vi "Initialize.vi"(6 "Actor Name":string, 7 "Host Name":string, 8 "error in (no error)":errorcluster, 11 "Message Broker":refnum<class "Message Broker Interface Ref.lvclass">) -> (0 "error out":errorcluster, 3 "User Interface out":refnum<class "User Interface.lvclass">)   [LabVIEW 2016, in "CLD Exam - ATM.lvlib" / "User Interface.lvclass"]
uses:
  User Interface.lvclass
  D:/Repos/Stream/software/Mediator/Classes/Mediated Actor/Mediated Actor.lvclass
  Mediator/Classes/Message Broker Interface Ref/Message Broker Interface Ref.lvclass
  D:/Repos/Stream/software/Mediator/Classes/Message Broker Interface/Message Broker Interface.lvclass
  Log/Application Log/Log Level.ctl
  Mediator/Classes/Message String/Message String.lvclass
  D:/Repos/Stream/software/Mediator/Classes/Message Interface/Message Interface.lvclass
  Mediator/Classes/Message Transport Queue/Message Transport Queue.lvclass
  D:/Repos/Stream/software/Mediator/Classes/Message Transport Interface/Message Transport Interface.lvclass
  Mediator/Classes/Mediated Actor/Mediated Actor.lvclass
  Log/Application Log/Application Log.lvclass
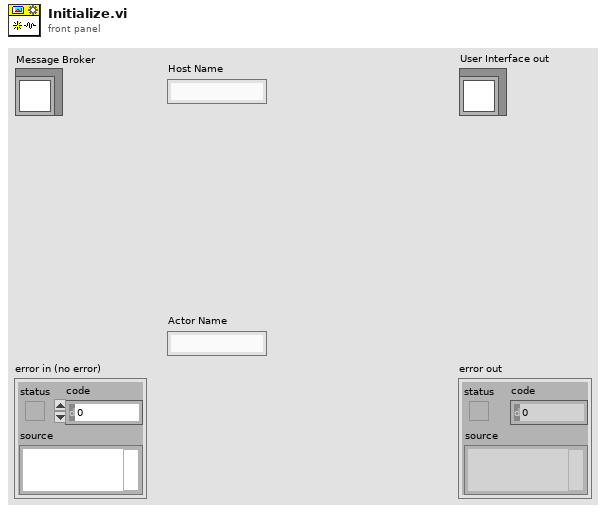
[diagram p1: front panel]
types:
  T1 = typedef "Stream Log.lvlib/Application Log.lvclass/Log Level.ctl" = enum16{"Imperative", "Major", "Minor", "Debug", "Off"}
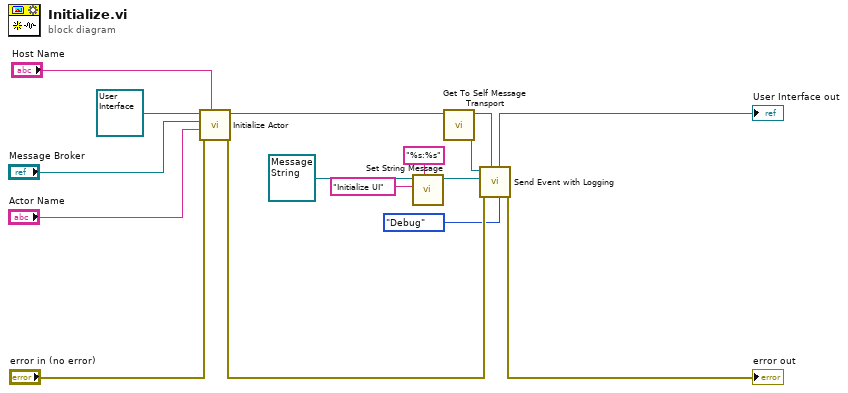
[diagram p0: block diagram]
diagram:
  n1 = call-dynamic "Initialize Actor.vi"("Host Name"="Host Name", "error in (no error)"="error in (no error)", "Actor Name"="Actor Name", "Message Broker Interface"="Message Broker", "User Interface in"=refnum<class "User Interface.lvclass"> refnum) -> ("error out"=w4:errorcluster, "User Interface out"=w10:refnum<class "User Interface.lvclass">)  [unwired: 5 in]
  n2 = call "Set String Message.vi"("Format"="%s:%s", "Name"="Initialize UI", "Message String in"=refnum<class "Message String.lvclass"> refnum ("Stream Mediator.lvlib:Message String.lvclass")) -> ("Message String out"=w5:refnum<class "Message String.lvclass">)  [unwired: 7 in, 1 out]
  n3 = call "Get To Self Message Transport.vi"("Mediated Actor in"=w10) -> ("To Self"=w6:refnum<class "Message Transport Queue.lvclass">, "Mediated Actor out"=w8:refnum<class "User Interface.lvclass">)  [unwired: 9 in]
  n4 = call "Send Event with Logging.vi"("Global Log Level"=Log_Level."Debug", "Mediated Actor in"=w8, "error in (no error)"=w4, "Message"=w5, "Message Transport Interface in"=w6) -> ("error out"=→"error out":errorcluster, "Mediated Actor out"=→"User Interface out":refnum<class "User Interface.lvclass">)  [unwired: 5 in]
